vi "Check Outgoing TP Timeouts.vi"(0 "J1939 Cluster":T7, 5 "Connection Refs":T1, 11 "error in":errorcluster) -> (13 "Message Error":errorcluster, 15 "error out":errorcluster)   [LabVIEW 2013, in "J1939 Addon Engine.lvlib"]
uses:
  Engine/J1939 Addon Engine.lvlib
  Types/Setup Information Cluster.ctl
  <vilib>/xnet/xnet.llb/XNET Frame CAN.ctl
  <vilib>/xnet/xnet.llb/XNET Frame Type CAN.ctl
  J1939 Utilities/Types/CAN Outgoing Message Cluster.ctl
  Types/TP List References.ctl
  Types/BAM Buffer Connections List_Ref.ctl
  Types/Connection Mode Generation Connection Ref.ctl
  Types/BAM Generation Connections List_Ref.ctl
  Types/Address Table Reference.ctl
  Types/RQST Lookup Table Reference.ctl
  J1939 Multi Packet Frames/Connection Mode Generation.vi
  SubVIs/Connection Mode Generation Connections List_Actions.vi
  SubVIs/Connection Mode Generation Get Next Messages.vi
  J1939 Utilities/SubVIs/TP.Conn Abort.vi
  J1939 Utilities/Common Conversions.vi
  J1939 Utilities/SubVIs/Convert J1939 ID to CAN Arb ID.vi
  J1939 Utilities/J1939 Utilities.lvlib
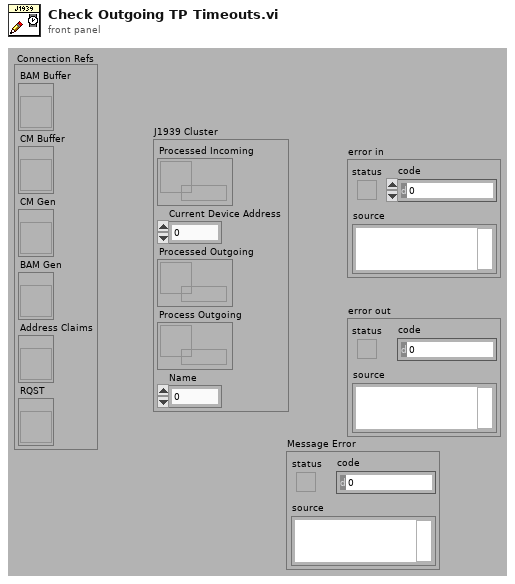
[diagram p1: front panel]
types:
  T1 = typedef "J1939 Addon Engine.lvlib/TP List References.ctl" = cluster{"BAM Buffer":T2, "CM Buffer":T2, "CM Gen":T3, "BAM Gen":T4, "Address Claims":T5, "RQST":T6}
  T2 = typedef "J1939 Addon Engine.lvlib/BAM Buffer Connections List_Ref.ctl" = refnum<vi>
  T3 = typedef "J1939 Addon Engine.lvlib/Connection Mode Generation Connection Ref.ctl" = refnum<vi>
  T4 = typedef "J1939 Addon Engine.lvlib/BAM Generation Connections List_Ref.ctl" = refnum<vi>
  T5 = typedef "J1939 Addon Engine.lvlib/Address Table Reference.ctl" = refnum<vi>
  T6 = typedef "J1939 Addon Engine.lvlib/RQST Lookup Table Reference.ctl" = refnum<vi>
  T7 = typedef "J1939 Addon Engine.lvlib/Setup Information Cluster.ctl" = cluster{"Processed Incoming":refnum<queue>, "Current Device Address":u8, "Processed Outgoing":refnum<queue>, "Process Outgoing":refnum<queue>, "Name":u64}
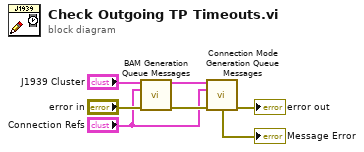
[diagram p0: block diagram]
diagram:
  n1 = call "BAM Generation Queue Messages.vi"("J1939 Cluster"="J1939 Cluster", "Connection Refs"="Connection Refs", "error in"="error in") -> ("J1939 Cluster Out"=w7:T7, "error out"=w6:errorcluster)  [unwired: 11 out]
  n2 = call "Connection Mode Generation Queue Messages.vi"("J1939 Cluster"=w7, "Connection Refs"="Connection Refs", "error in"=w6) -> ("Message Error"=→"Message Error":errorcluster, "System Error out"=→"error out":errorcluster)  [unwired: 11 out]
